vi "Make.vi"(8 "error in (no error)":errorcluster, 10 "Input":string) -> (0 "error out":errorcluster, 2 "map":map{string, refnum<class "Module.lvclass">}(c390), 3 "Proto":refnum<class "Module.lvclass">[](array[class]))   [LabVIEW 2021, in "Module.lvclass"]
uses:
  Module.lvclass
  Module.lvclass/Module.ctl
  Flip Flop/Flip Flop.lvclass
  C:/git/aoc-2023/Day 20/Proto/Module.lvclass
  Conjunction/Conjunction.lvclass
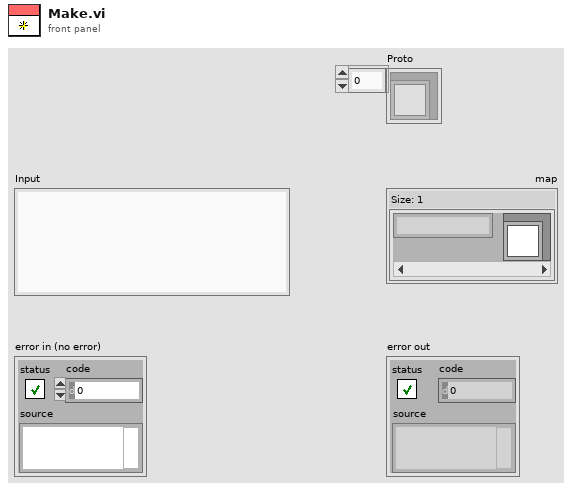
[diagram p1: front panel]
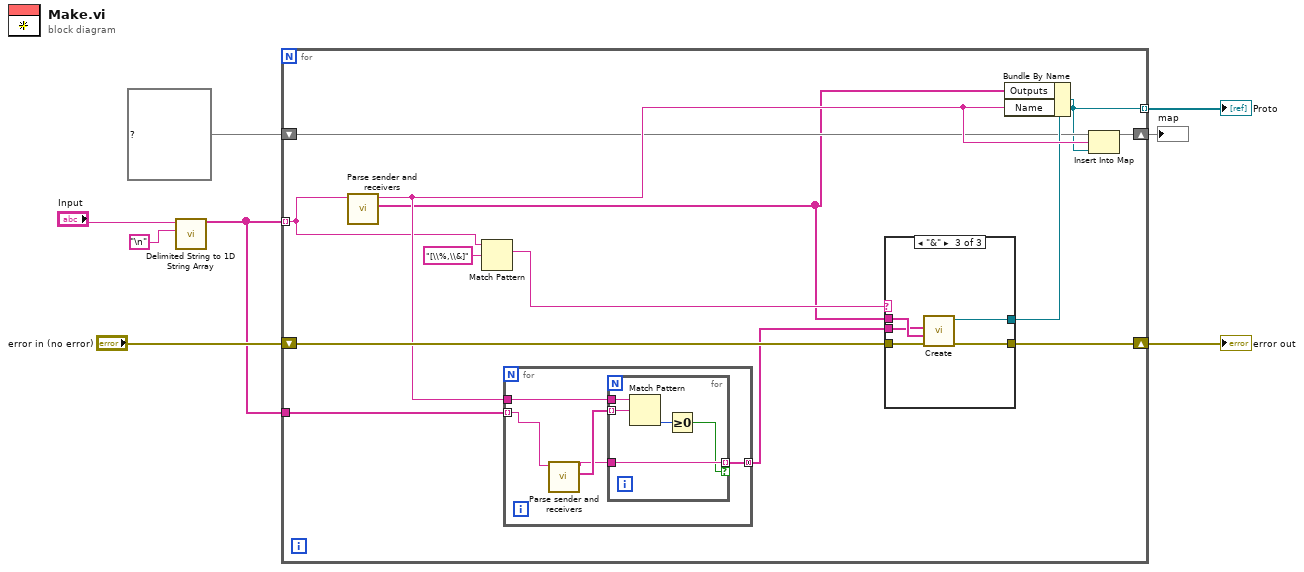
[diagram p0: block diagram]
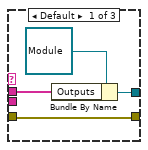
[diagram p2: hidden frame]
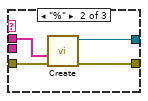
[diagram p3: hidden frame]
diagram:
  n1 = call <vilib>:"Delimited String to 1D String Array.vi"("delimiter"="\n", "delimited string"="Input") -> ("string array"=w3:string[])  [unwired: 9 in]
  n2 = for {
    tunnel: [w10] -> w6 mode=indexing
    tunnel: w3 -> [w12] mode=indexing
    shift-right: [w20] -> w7
    shift-left: "error in (no error)" -> [w21]
    tunnel: w3 -> [w19]
    shift-right: [w14] -> w1
    shift-left: map{string, refnum<class "Module.lvclass">} {} ("map") -> [w15]
    n3 = call "Parse sender and receivers.vi"("String"=w12) -> ("Receivers"=w9:string[], "Sender"=w17:string)  [unwired: 9 in]
    n4 = Match Pattern(string=w12, regular expression="[\\%,\\&]") -> (match substring=w11:string)  [unwired: 1 in, 3 out]
    n5 = for {
      tunnel: w19 -> [w25] mode=indexing
      tunnel: w17 -> [w26]
      tunnel: [w22] -> w18 mode=concatenating
      n6 = call "Parse sender and receivers.vi"("String"=w25) -> ("Receivers"=w24:string[], "Sender"=w23:string)  [unwired: 9 in]
      n7 = for {
        tunnel: w26 -> [w31]
        tunnel: w24 -> [w30] mode=indexing
        tunnel: w23 -> [w28]
        tunnel: [w28] -> w22 mode=indexing if=w27
        n8 = Match Pattern(string=w31, regular expression=w30) -> (offset past match=w29:i32)  [unwired: 1 in, 3 out]
        n9 = Greater Or Equal To 0?(x=w29) -> (x >= 0?=w27:bool)
      }
    }
    n10 = case shown="\"&\"" w11 {
      tunnel: w21 -> [w32 w39 w44]
      tunnel: [w32 w38 w43] -> w20
      tunnel: w9 -> [w34 w37 w42]
      tunnel: [w33 w36 w41] -> w16
      tunnel: w18 -> [_ _ w40]
      frame Default {
        n11 = Bundle By Name(cluster=refnum<class "Module.lvclass"> refnum ("Module.lvclass"), "Outputs"=w34) -> (w33:refnum<class "Module.lvclass">)
      }
      frame "%" {
        n12 = call "Create.vi"("error in (no error)"=w39, "Outputs"=w37) -> ("error out"=w38:errorcluster, "Flip Flop"=w36:refnum<class "Flip Flop.lvclass">)  [unwired: 8 in]
      }
      frame "&" {
        n13 = call "Create.vi"("error in (no error)"=w44, "Outputs"=w42, "Inputs"=w40) -> ("error out"=w43:errorcluster, "Conjunction"=w41:refnum<class "Conjunction.lvclass">)  [unwired: 7 in]
      }
    }
    n14 = Bundle By Name(cluster=w16, "Outputs"=w9, "Name"=w17) -> (w10:refnum<class "Module.lvclass">)
    n15 = Insert Into Map(map in=w15, key=w17, value=w10) -> (map out=w14:map{string, refnum<class "Module.lvclass">})  [unwired: 2 out]
  }
  "error out" <- w7
  "Proto" <- w6
  "map" <- w1
